vi "Trav_3D_volume.vi"(3 "Simulate/Run":T1, 5 "Traverse line":T2 {"Row Duration (mins)" format="%#.1f"; "Row No" min=0; "Trace Gas Concentration (%)" min=0.0 format="%#.2f"; "Emission Rate (l/min)" format="%#.2f"; "Tunnel Speed" format="%#.2f"; "Start X" format="%#.2f"; "Start Y" format="%#.2f"; "Start Z" format="%#.2f"; "End X" format="%#.2f"; "End Y" format="%#.2f"; "End Z" format="%#.2f"; "Averaging time (min)" min=0.0 format="%#.2f"}) -> (0 "Error Messages":string, 1 "Status":T5, 2 "Traverse line Out":T2 {"Row Duration (mins)" format="%#.1f"; "Row No" min=0; "Trace Gas Concentration (%)" min=0.0 format="%#.2f"; "Emission Rate (l/min)" format="%#.2f"; "Tunnel Speed" format="%#.2f"; "Start X" format="%#.2f"; "Start Y" format="%#.2f"; "Start Z" format="%#.2f"; "End X" format="%#.2f"; "End Y" format="%#.2f"; "End Z" format="%#.2f"; "Averaging time (min)" min=0.0 format="%#.2f"})   [LabVIEW 2011]
uses:
  Gen Trav/Multi_Run_Status.ctl
  Gen Trav/Traverse_cluster.ctl
  Gen Trav/Spacing.ctl
  Controls/Multi_run_mode.ctl
  Controls/User_Specific_mode.ctl
  Controls/Save_Data.ctl
  Controls/Setup.ctl
  ADAM Client/Sub VIs/ADAM Controls/Traverse_Level_State.ctl
  Controls/Overhead.ctl
  Globals/Trav_pos_global.vi
  Globals/Meas_global.vi
panel:
  out "Pause message":string
  in  "Pause":bool
  out "Current position":dbl[](array[numeric]) format="%.2f"
  in  "stop":bool
  in  "Array of Positions":dbl[][](array[numeric]) format="%.2f"
  out "Abcissa copy":string="Y (mm)"
  out "Abcissa":string="Y (mm)"
  in  "Plot 1":i32[](listbox)=[1]
  out "Started Profile at:":string="16/9/98 12:33"
  out "Currently on point":i32=9
  out "U":cluster{dbl[], dbl[]}[](graph)
  out "% u'/U":cluster{dbl[], dbl[]}[](graph)
  # "X           Y            Z"
  # "Start"
  # "End"
  # "X           Y            Z"
  # "Start"
  # "End"
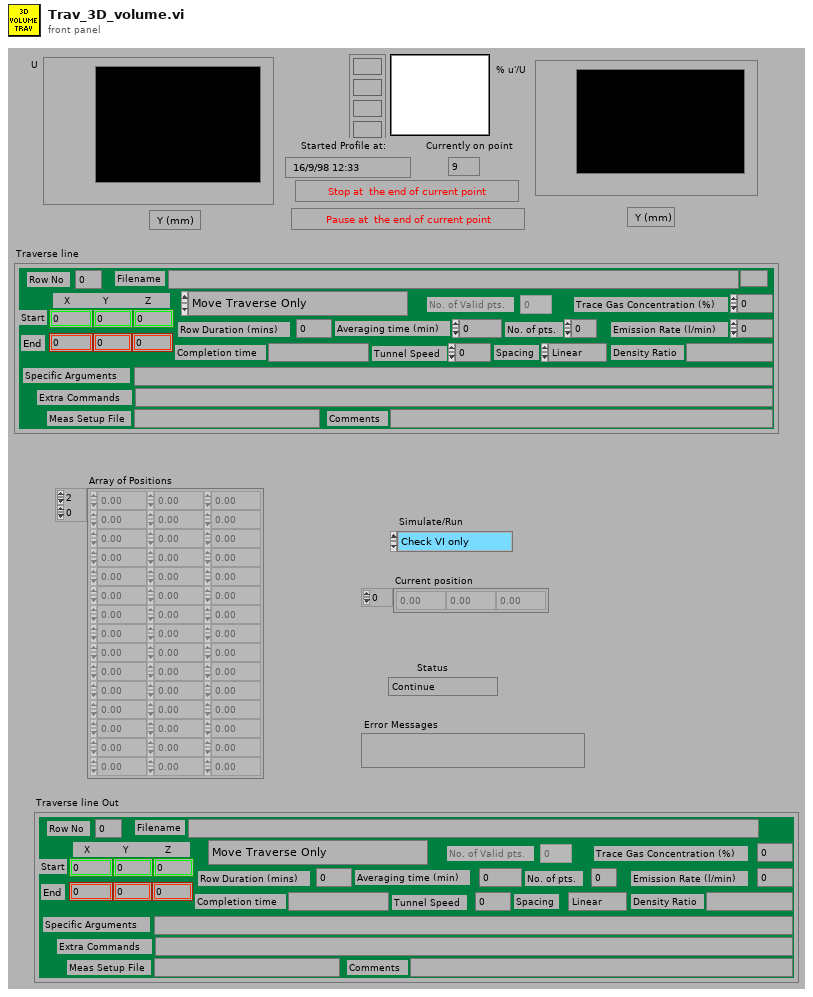
[diagram p1: front panel]
types:
  T1 = typedef "User_Specific_mode.ctl" = enum16{"Check VI only", "Run VI"}
  T2 = typedef "Traverse_cluster.ctl" = cluster{"Start X":dbl, "Start Y":dbl, "Start Z":dbl, "End X":dbl, "End Y":dbl, "End Z":dbl, "No. of pts.":i32, "Spacing":T3, "Filename":path, "Tunnel Speed":dbl, "Averaging time (min)":dbl, "Extra Commands":string, "Specific Arguments":string, "Emission Rate (l/min)":dbl, "Trace Gas Concentration (%)":dbl, "Density Ratio":string, "Comments":string, "Row No":i32, "Row Type Selector":T4, "Completion time":string, "Row Duration (mins)":dbl, "No. of Valid pts.":i32, "Meas Setup File":string}
  T3 = typedef "Spacing.ctl" = enum16{"Linear", "Log", "Gauss", "Specified", "N/A"}
  T4 = typedef "Multi_run_mode.ctl" = enum16{"Move Traverse Only", "Set Tunnel Speed Only", "Set Source Only", "Set Measurement Conditions", "Single Measurement", "Vertical Profile", "Lateral Profile", "Longitudinal Profile", "Explore Volume", "Multi-Axis Profile", "Auto Calibrate", "Meas Fast FID Bkgnd", "Check Beam Power", "Scanning Valve Measurement", "Run VI Named:", "Set ADAM Ch", "Wait (minutes)", "Send Message", "Synchronize With:", "Fall Back to this Row", "Turn Off Row Repeating", "Blank Row", "Traverse 3D Volume"}
  T5 = typedef "Multi_Run_Status.ctl" = enum16{"Continue", "Jump to Next Point", "Jump to Next Row", "Jump To Fall Back", "Terminate Run"}
  T6 = typedef "Save_Data.ctl" = enum16{"Save No Data", "Save Data"}
  T7 = typedef "Setup.ctl" = enum16{"Run Program", "Show Setup", "Save Current Setup", "Setup Front Panel"}
  T8 = typedef "Traverse_Level_State.ctl" = enum16{"Running", "Complete"}
  T9 = typedef "Overhead.ctl" = enum16{"Update total times", "Read Current Overhead", "Re Scale totals to 3 hrs", "Initialise totals to 3hr"}
  T10 = typedef "Status_Cluster.ctl" = cluster{"Status":T5, "Error Type":string, "Error Description":string}
  T11 = typedef "Analysis_info_cluster.ctl" = cluster{"Colour":u32, "Inst type":T12, "Inst name":string, "Symbol":string, "Code name":string, "Extra Info":string, "Inst Array":T13, "Extra Titles":string[], "Extra Values":string[], "Eng Values":dbl[], "Time (ms)":dbl[], "Voltage":dbl[], "U":dbl, "u^2":dbl, "u^3":dbl, "u^4":dbl, "Skew_u":dbl, "Kurt_u":dbl, "Sd Error in Mean":dbl, "% u'/U":dbl, "X":dbl, "Y":dbl, "Z":dbl, "Spectra":T14, "Autocorrelation":T14, "Timescale integral to 25%":dbl, "Sd Error in Variance":dbl, "Calib File":path, "Calib Constants":dbl[], "Histogram":T14, "Output Position":bool, "Full Stats":bool, "Weighting":dbl[], "Av Sampling Rate":dbl, "Av No of Samples":dbl, "Total Meas Time (s)":dbl, "ADAM Ch Name":string}
  T12 = typedef "Inst_type.ctl" = enum16{"Propeller anemometer", "Raw voltage", "Pressure Transducer", "Pitot-static tube", "Preston tube", "Hot wire", "Cross wire 1", "Cross wire 2", "Generic Linear", "Generic Polynomial", "Generic BackPoly", "Fast FID", "Thermocouple", "Cold wire", "Pulsed Wire", "LDA Vel", "LDA Tran time", "LDA Arr time"}
  T13 = typedef "Instrument_Array.ctl" = enum16{"PWA", "LDA", "Analogue"}
  T14 = typedef "XY_Plot_Cluster.ctl" = cluster{"First Name":string, "Second Name":string, "X axis name":string, "Y axis name":string, "X array":dbl[], "Y array":dbl[]}
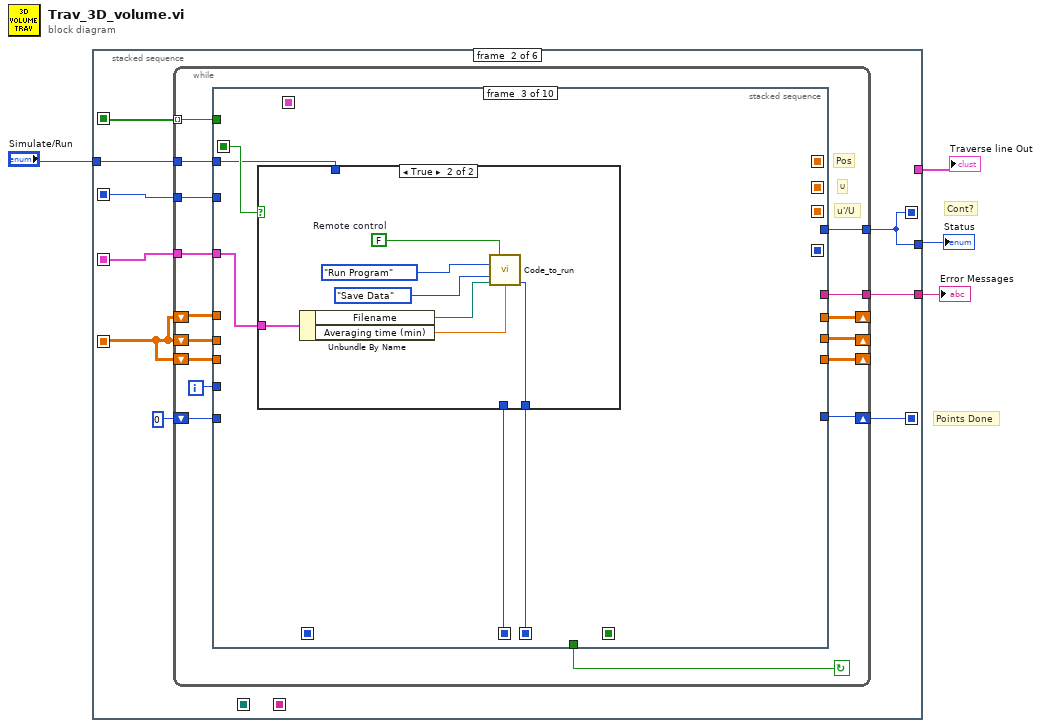
[diagram p0: block diagram]
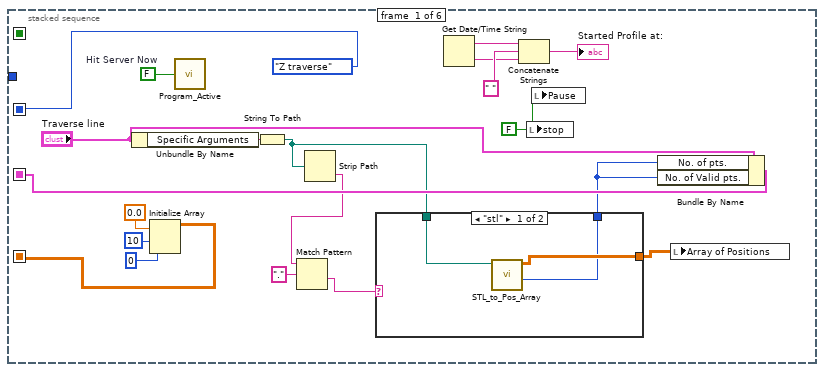
[diagram p2: hidden frame]
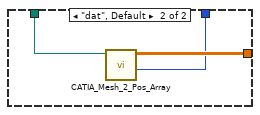
[diagram p3: hidden frame]
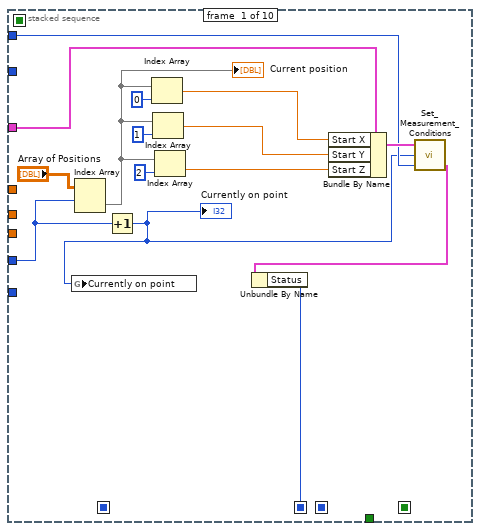
[diagram p4: hidden frame]
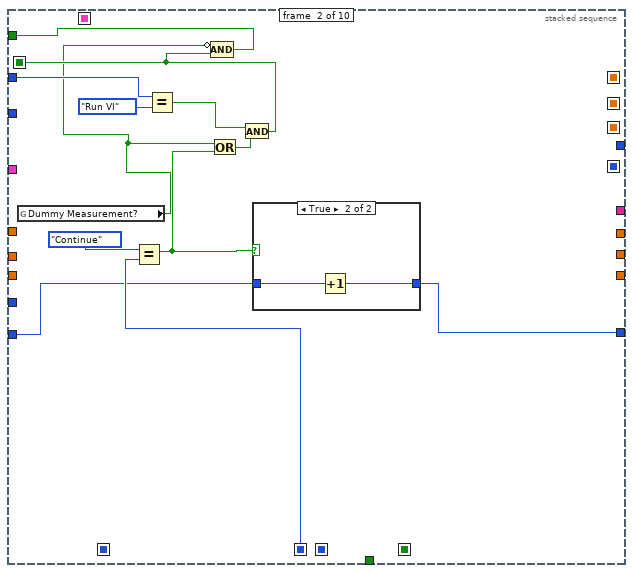
[diagram p5: hidden frame]
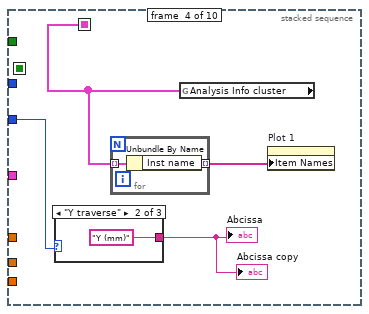
[diagram p8: hidden frame]
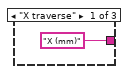
[diagram p9: hidden frame]
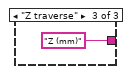
[diagram p10: hidden frame]
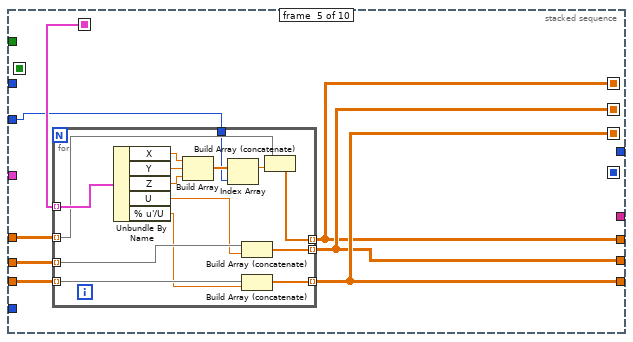
[diagram p11: hidden frame]
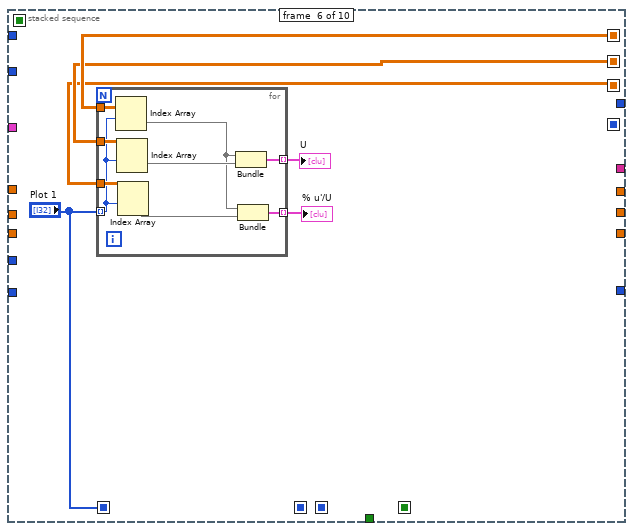
[diagram p12: hidden frame]
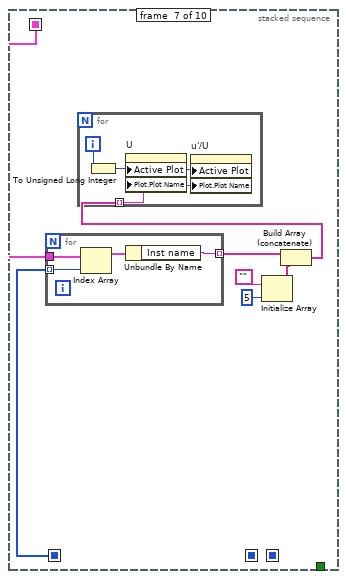
[diagram p13: hidden frame]
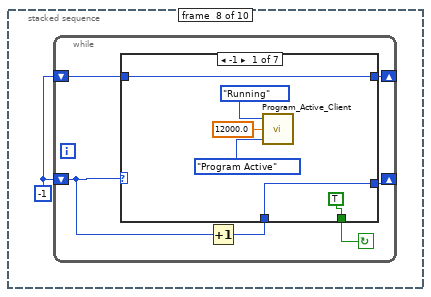
[diagram p14: hidden frame]
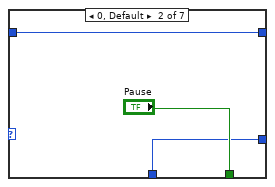
[diagram p15: hidden frame]
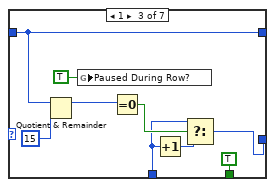
[diagram p16: hidden frame]
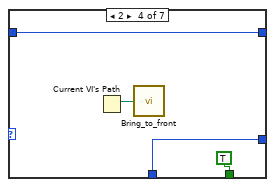
[diagram p17: hidden frame]
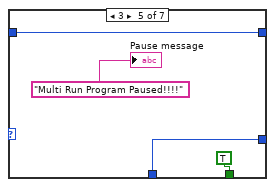
[diagram p18: hidden frame]
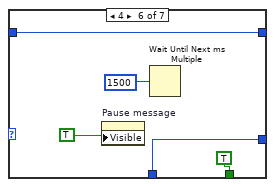
[diagram p19: hidden frame]
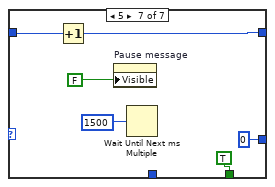
[diagram p20: hidden frame]
diagram:
  # "Points Done"
  # "Cont?"
  n1 = stacked-sequence {
    seq-local: [w17 _ _ _ _ _] -> [_ w38 _ _ _ _]
    seq-local: [enum16{"X traverse", "Y traverse", "Z traverse"}."Z traverse" ("Axis Traversed") _ _ _ _ _] -> [_ w39 _ _ _ _]
    seq-local: [_ _ w264 _ _ _] -> [_ _ _ _ w288 _]
    seq-local: [_ _ _ w271 _ _] -> [_ _ _ _ w287 _]
    seq-local: [_ w37 _ _ _ _] -> [_ _ _ _ _ _]
    seq-local: [_ w35 _ _ _ _] -> [_ _ _ w268 w286 _]
    seq-local: [_ w33 _ _ _ _] -> [_ _ _ _ _ w293]
    seq-local: [w10 _ _ _ _ _] -> [_ w32 _ _ _ w295]
    tunnel: [_ w37 _ _ _ _] -> w2
    tunnel: [_ _ _ _ _ w305] -> w4
    tunnel: "Simulate/Run" -> [_ w36 _ _ _ w304]
    tunnel: [_ w31 _ _ _ _] -> w1
    frame #0 {
      w15 = FALSE ("stop")
      w16 = FALSE  # Hit Server Now
      n2 = Unbundle By Name("Traverse line") -> ("Specific Arguments"=w12:string)
      n3 = Initialize Array(0.0, 10, 0) -> (w17:dbl[][])
      n4 = call "Program_Active.vi"("Hit Server Now"=w16) -> ()
      n5 = String To Path(string=w12) -> (path=w8:path)
      n6 = Strip Path(path=w8) -> (name=w6:string)  [unwired: 1 out]
      n7 = Match Pattern(string=w6, regular expression=".") -> (after substring=w5:string)  [unwired: 1 in, 3 out]
      n8 = case shown="\"stl\"" w5 {
        tunnel: [w26 w30] -> w13
        tunnel: [w25 w29] -> w9
        tunnel: w8 -> [w27 w28]
        frame "stl" {
          n9 = call "STL_to_Pos_Array.vi"("STL file"=w27) -> ("Number of Points"=w25:i32, "Array of Positions"=w26:dbl[][])  [unwired: 9 in]
        }
        frame "dat", Default {
          n10 = call "CATIA_Mesh_2_Pos_Array.vi"("Catia Mesh File"=w28) -> ("Number of Points"=w29:i32, "Array of Positions"=w30:dbl[][])  [unwired: 9 in]
        }
      }
      n11 = Get Date/Time String() -> (date string=w23:string, time string=w22:string)  [unwired: 3 out]
      n12 = Concatenate Strings(w23, " ", w22) -> (→"Started Profile at:":string)
      n13 = local write "stop"(w15) -> ()
      n14 = local write "Pause"(w15) -> ()
      n15 = Bundle By Name(cluster="Traverse line", "No. of pts."=w9, "No. of Valid pts."=w9) -> (w10:T2)
      n16 = local write "Array of Positions"(w13) -> ()
    }
    frame #1 {
      n17 = while {
        shift-left: 0 -> [w42]
        shift-right: [w41] -> w33
        tunnel: [w43] -> w35 mode=indexing
        tunnel: w32 -> [w44]
        tunnel: w36 -> [w45]
        tunnel: [w46] -> w37
        shift-left: w38 -> [w49]
        shift-right: [w48] -> _
        tunnel: w39 -> [w50]
        shift-left: w38 -> [w52]
        shift-right: [w51] -> _
        shift-left: w38 -> [w54]
        shift-right: [w53] -> _
        tunnel: [w40] -> w31
        i -> [w55]
        stop <- w47 continue-if-true
        # "Pos"
        # "U"
        # "u'/U"
        n18 = stacked-sequence {
          seq-local: [_ _ _ w102 _ _ _ _ _ _] -> [_ _ _ _ w113 _ w146 _ _ _]
          seq-local: [_ _ _ _ w109 _ _ _ _ _] -> [_ _ _ _ _ w136 _ _ _ _]
          seq-local: [_ _ _ _ w111 _ _ _ _ _] -> [_ _ _ _ _ w135 _ _ _ _]
          seq-local: [_ _ _ _ w112 _ _ _ _ _] -> [_ _ _ _ _ w134 _ _ _ _]
          seq-local: [_ _ _ _ _ "Plot 1" _ _ _ _] -> [_ _ _ _ _ _ w152 _ _ _]
          seq-local: [_ _ w89 _ _ _ _ _ _ _] -> [_ _ _ _ _ _ _ _ w210 _]
          seq-local: [w60 _ _ _ _ _ _ _ _ _] -> [_ w80 w87 _ _ _ _ _ _ _]
          seq-local: [_ w73 _ _ _ _ _ _ _ _] -> [_ _ w88 _ _ _ _ _ _ _]
          seq-local: [_ _ _ _ _ _ _ _ w205 _] -> [_ _ _ _ _ _ _ _ _ w226]
          seq-local: [_ _ _ _ _ _ _ _ w204 _] -> [_ _ _ _ _ _ _ _ _ w220]
          tunnel: w55 -> [w57 _ _ _ _ _ _ _ w216 w223]
          tunnel: w54 -> [_ _ _ _ w115 _ _ _ _ _]
          tunnel: [_ _ _ _ w111 _ _ _ _ _] -> w53
          tunnel: w52 -> [_ _ _ _ w114 _ _ _ _ _]
          tunnel: [_ _ _ _ w112 _ _ _ _ _] -> w51
          tunnel: w50 -> [_ _ _ w100 w108 _ _ _ _ _]
          tunnel: w49 -> [_ _ _ _ w110 _ _ _ _ _]
          tunnel: [_ _ _ _ w109 _ _ _ _ _] -> w48
          tunnel: [_ _ _ _ _ _ _ _ w205 _] -> w47
          tunnel: w44 -> [w64 _ w90 _ _ _ _ _ _ w224]
          tunnel: [_ _ _ _ _ _ _ _ _ w222] -> w46
          tunnel: w45 -> [w62 w82 w86 _ _ _ _ _ _ w225]
          tunnel: [_ w72 _ _ _ _ _ _ _ _] -> w43
          tunnel: w42 -> [_ w77 _ _ _ _ _ _ _ _]
          tunnel: [_ w76 _ _ _ _ _ _ _ _] -> w41
          tunnel: [_ _ _ _ _ _ _ _ _ w221] -> w40
          frame #0 {
            n19 = Index Array(array="Array of Positions", index (row)=w57) -> (element=w56:dbl[])  [unwired: 1 in]
            "Current position" <- w56
            n20 = Increment(x=w57) -> (x+1=w59:i32)
            "Currently on point" <- w59
            n21 = global write "Trav_pos_global.vi" "Currently on point"(w59) -> ()
            n22 = Index Array(array=w56, index=0 ("Index")) -> (element=w67:dbl)
            n23 = Index Array(array=w56, index=1 ("Index")) -> (element=w66:dbl)
            n24 = Index Array(array=w56, index=2 ("Index")) -> (element=w65:dbl)
            n25 = Bundle By Name(cluster=w64, "Start X"=w67, "Start Y"=w66, "Start Z"=w65) -> (w63:T2)
            n26 = call "Set_Measurement_Conditions.vi"("Simulate/Run"=w62, "Currently on Point"=w59, "Traverse line"=w63) -> ("Status Cluster"=w61:T10)  [unwired: 2 out]
            n27 = Unbundle By Name(w61) -> ("Status"=w60:T5)
          }
          frame #1 {
            n28 = global read "Trav_pos_global.vi" "Dummy Measurement?"() -> (w71:bool)
            n29 = Equal?(x=Multi_Run_Status."Continue" ("Status"), y=w80) -> (x = y?=w75:bool)
            n30 = Equal?(x=w82, y=User_Specific_mode."Run VI" ("Simulate/Run")) -> (x = y?=w78:bool)
            n31 = Or(x=w71, y=w75) -> (x .or. y?=w74:bool)
            n32 = And(x=w78, y=w74) -> (x .and. y?=w73:bool)
            n33 = Compound Arithmetic op=AND(invert w71, w73) -> (w72:bool)
            n34 = case shown="True" w75 {
              tunnel: w77 -> [w83 w85]
              tunnel: [w83 w84] -> w76
              frame False {
              }
              frame True {
                n35 = Increment(x=w85) -> (x+1=w84:i32)
              }
            }
          }
          frame #2 {
            n36 = case shown="True" w88 {
              tunnel: w90 -> [_ w98]
              tunnel: [w91 w97] -> w89
              tunnel: w87 -> [w91 _]
              tunnel: w86 -> [_ _]
              frame False {
              }
              frame True {
                w96 = FALSE  # Remote control
                n37 = Unbundle By Name(w98) -> ("Filename"=w94:path, "Averaging time (min)"=w95:dbl)
                n38 = call "Code_to_run.vi"("setup"=Setup."Run Program", "Remote control"=w96, "File"=Save_Data."Save Data", "Results Filename"=w94, "Averaging time (min)"=w95) -> ("Status"=w97:T5)  [unwired: 6 in, 4 out]
              }
            }
          }
          frame #3 {
            n39 = case shown="\"Y traverse\"" w100 {
              tunnel: ["X (mm)" "Y (mm)" "Z (mm)"] -> w99
              frame "X traverse" {
              }
              frame "Y traverse" {
              }
              frame "Z traverse" {
              }
            }
            "Abcissa" <- w99
            "Abcissa copy" <- w99
            n40 = global read "Meas_global.vi" "Analysis Info cluster"() -> (w102:T11[])
            n41 = for {
              tunnel: w102 -> [w107] mode=indexing
              tunnel: [w106] -> w101 mode=indexing
              n42 = Unbundle By Name(w107) -> ("Inst name"=w106:string)
            }
            n43 = property on="Plot 1" class="LstBox (strict)"("Item Names"=w101) -> ()  [unwired: 2 in, 2 out]
          }
          frame #4 {
            n44 = for {
              tunnel: w115 -> [w130] mode=indexing
              tunnel: [w128] -> w111 mode=indexing
              tunnel: w114 -> [w127] mode=indexing
              tunnel: [w125] -> w112 mode=indexing
              tunnel: w113 -> [w124] mode=indexing
              tunnel: w110 -> [w123] mode=indexing
              tunnel: [w122] -> w109 mode=indexing
              tunnel: w108 -> [w117]
              n45 = Unbundle By Name(w124) -> ("X"=w121:dbl, "Y"=w120:dbl, "Z"=w119:dbl, "U"=w129:dbl, "% u'/U"=w126:dbl)
              n46 = Build Array(w121, w120, w119) -> (w118:dbl[])
              n47 = Index Array(array=w118, index=w117) -> (element=w116:dbl)
              n48 = Build Array (concatenate)(w130, w129) -> (w128:dbl[])
              n49 = Build Array (concatenate)(w127, w126) -> (w125:dbl[])
              n50 = Build Array (concatenate)(w123, w116) -> (w122:dbl[])
            }
          }
          frame #5 {
            n51 = for {
              tunnel: "Plot 1" -> [w137] mode=indexing
              tunnel: w136 -> [w145]
              tunnel: w135 -> [w144]
              tunnel: w134 -> [w143]
              tunnel: [w139] -> w133 mode=indexing
              tunnel: [w138] -> w132 mode=indexing
              n52 = Index Array(array=w145, index (row)=w137) -> (element=w141:dbl[])  [unwired: 1 in]
              n53 = Index Array(array=w144, index (row)=w137) -> (element=w142:dbl[])  [unwired: 1 in]
              n54 = Index Array(array=w143, index (row)=w137) -> (element=w140:dbl[])  [unwired: 1 in]
              n55 = Bundle(w141, w142) -> (w138:cluster{dbl[], dbl[]})  [unwired: 1 out]
              n56 = Bundle(w141, w140) -> (w139:cluster{dbl[], dbl[]})  [unwired: 1 out]
            }
            "U" <- w132
            "% u'/U" <- w133
          }
          frame #6 {
            n57 = for {
              tunnel: w152 -> [w156] mode=indexing
              tunnel: w146 -> [w154]
              tunnel: [w153] -> w149 mode=indexing
              n58 = Index Array(array=w154, index=w156) -> (element=w155:T11)
              n59 = Unbundle By Name(w155) -> ("Inst name"=w153:string)
            }
            n60 = Initialize Array("", 5) -> (w148:string[])
            n61 = Build Array (concatenate)(w149, w148) -> (w147:string[])
            n62 = for {
              tunnel: w147 -> [w157] mode=indexing
              i -> [w159]
              n63 = To Unsigned Long Integer(number=w159) -> (unsigned 32bit integer=w158:u32)
              n64 = property on="U" class="XYGraph (strict)"("Active Plot"=w158, "Plot.Plot Name"=w157) -> ()  [unwired: 2 in, 2 out]
              n65 = property on="u'/U" class="XYGraph (strict)"("Active Plot"=w158, "Plot.Plot Name"=w157) -> ()  [unwired: 2 in, 2 out]
            }
          }
          frame #7 {
            w160 = -1
            n66 = while {
              shift-left: w160 -> [w161]
              shift-right: [w162] -> _
              shift-left: w160 -> [w165]
              shift-right: [w166] -> _
              stop <- w163 continue-if-true
              n67 = Increment(x=w165) -> (x+1=w164:i32)
              n68 = case shown="-1" w165 {
                tunnel: [w171 w174 w178 w188 w191 w195 0] -> w166
                tunnel: w164 -> [w171 w174 w180 w188 w191 w195 _]
                tunnel: [TRUE ("Pause") "Pause" TRUE ("Pause") TRUE ("Pause") TRUE ("Pause") TRUE ("Pause") TRUE ("Pause")] -> w163
                tunnel: [w170 w173 w176 w185 w189 w193 w198] -> w162
                tunnel: w161 -> [w170 w173 w176 w185 w189 w193 w199]
                frame -1 {
                  n69 = call "Program_Active_Client.vi"("Mode"=enum16{"Program Active", "Traverse Level State"}."Program Active", "Time till next contact (Sec)"=12000.0, "Traverse level State"=Traverse_Level_State."Running") -> ()  [unwired: 3 out]
                }
                frame 0, Default {
                }
                frame 1 {
                  n70 = Quotient & Remainder(x=w176, y=15) -> (x-y*floor(x/y)=w182:i32)  [unwired: 1 out]
                  n71 = global write "Trav_pos_global.vi" "Paused During Row?"(TRUE ("Paused During Row?")) -> ()
                  n72 = Equal To 0?(x=w182) -> (x = 0?=w181:bool)
                  n73 = Increment(x=w180) -> (x+1=w179:i32)
                  n74 = Select(t=w180, s=w181, f=w179) -> (s? t:f=w178:i32)
                }
                frame 2 {
                  n75 = Current VI's Path() -> (path=w186:path)
                  n76 = call "Bring_to_front.vi"("path"=w186) -> ()
                }
                frame 3 {
                  "Pause message" <- "Multi Run Program Paused!!!!" ("Pause message")
                }
                frame 4 {
                  n77 = property on="Pause message" class="Str"("Visible"=TRUE) -> ()  [unwired: 2 in, 2 out]
                  n78 = Wait Until Next ms Multiple(millisecond multiple=u32 1500) -> ()  [unwired: 1 out]
                }
                frame 5 {
                  n79 = Increment(x=w199) -> (x+1=w198:i32)
                  n80 = property on="Pause message" class="Str"("Visible"=FALSE) -> ()  [unwired: 2 in, 2 out]
                  n81 = Wait Until Next ms Multiple(millisecond multiple=u32 1500) -> ()  [unwired: 1 out]
                }
              }
            }
          }
          frame #8 {
            n82 = Increment(x=w216) -> (x+1=w215:i32)
            n83 = local read "Array of Positions"() -> (w206:dbl[][])
            n84 = case shown="\"Jump to Next Point\"" w210 {
              tunnel: [TRUE TRUE FALSE] -> w213
              frame "Continue" {
              }
              frame "Jump to Next Point" {
              }
              frame "Jump to Next Row", Default {
              }
            }
            n85 = Array Size(array=w206) -> (size(s)=w209:i32[])
            n86 = Index Array(array=w209, index=0 ("Index")) -> (element=w207:i32)
            n87 = Less?(x=w215, y=w207) -> (x < y?=w214:bool)
            n88 = Compound Arithmetic op=AND(w213, invert "stop", w214) -> (w205:bool)
            n89 = Select(t=Multi_Run_Status."Terminate Run" ("Status"), s="stop", f=w210) -> (s? t:f=w204:T5)
          }
          frame #9 {
            n90 = case shown="True" w226 {
              tunnel: w225 -> [_ w235]
              tunnel: w224 -> [_ w234]
              tunnel: w223 -> [_ w233]
              tunnel: [w228 w230] -> w222
              tunnel: ["" w229] -> w221
              tunnel: w220 -> [w228 _]
              frame False {
              }
              frame True {
                n91 = case shown="\"Check VI only\"" w235 {
                  tunnel: w234 -> [w251 _]
                  tunnel: w233 -> [w246 _]
                  tunnel: [w236 timestamp(0 s since 1904-01-01)] -> w232
                  frame "Check VI only" {
                    n92 = Increment(x=w246) -> (x+1=w244:i32)
                    n93 = Unbundle By Name(w251) -> ("Averaging time (min)"=w248:dbl)
                    n94 = global read "Trav_pos_global.vi" "Simulation Time"() -> (w238:timestamp)
                    n95 = To Double Precision Float(number=w238) -> (double precision float=w239:dbl)
                    n96 = Multiply(x=60.0, y=w248) -> (x*y=w247:dbl)
                    n97 = Add(x=w247, y=10.0 ("Scalable Time (Sec)")) -> (x+y=w245:dbl)
                    n98 = Multiply(x=w245, y=w244) -> (x*y=w242:dbl)
                    n99 = call "Overhead_Factor.vi"("Mode"=Overhead."Read Current Overhead") -> ("Current Overhead Factor"=w243:dbl)  [unwired: 3 in]
                    n100 = Multiply(x=w243, y=w242) -> (x*y=w240:dbl)
                    n101 = Add(x=w239, y=w240) -> (x+y=w237:dbl)
                    n102 = To Time Stamp(1:w237) -> (0:w236:timestamp)
                  }
                  frame "Run VI" {
                  }
                }
                n103 = call "Run_FFID_Bkgnd.vi"("Simulated Time"=w232, "Run Now?"=FALSE, "Simulate/Run"=w235) -> ("Error Messages"=w229:string, "Status"=w230:T5)  [unwired: 1 out]
              }
            }
          }
        }
      }
    }
    frame #2 {
      n104 = global read "Meas_global.vi" "Start Time of experiment"() -> (w254:dbl)
      n105 = global read "Meas_global.vi" "Raw data file"() -> (w266:path)
      n106 = Strip Path(path=w266) -> (stripped path=w265:path)  [unwired: 1 out]
      n107 = call "Sec_to_date_filename.vi"("seconds"=w254) -> ("Day"=w256:string, "Time"=w257:string)  [unwired: 2 out]
      n108 = Format Into String(format string="Cmd_%s_%s.xls", w256, w257) -> (resulting string=w259:string)  [unwired: 2 in, 1 out]
      n109 = call "Fast_string_Replace.vi"("Replace match with:"="-", "Input String"=w259, "regular expression"=":") -> ("Output String"=w262:string)  [unwired: 2 out]
      n110 = call "Fast_string_Replace.vi"("Replace match with:"="", "Input String"=w262, "regular expression"=" ") -> ("Output String"=w253:string)  [unwired: 2 out]
      n111 = Build Path(base path=w265, name or relative path=w253) -> (appended path=w264:path)
    }
    frame #3 {
      w277 = "\t"
      n112 = local read "Array of Positions"() -> (w270:dbl[][])
      n113 = Number To Fractional String(number=w270, precision (6)=i16 2) -> (F-format string=w269:string[][])  [unwired: 2 out]
      n114 = for {
        tunnel: w269 -> [w282] mode=indexing
        tunnel: w268 -> [w281] mode=indexing
        tunnel: [w279] -> w267 mode=indexing
        n115 = case shown="False" w281 {
          tunnel: ["Unobtainable Position" ""] -> w280
          frame False {
          }
          frame True {
          }
        }
        n116 = Build Array (concatenate)(w282, w280) -> (w279:string[])
      }
      n117 = Concatenate Strings("X", w277, "Y", w277, "Z") -> (w272:string)
      n118 = call "2D_array_to_string.vi"("2D data array"=w267, "Column titles  (separated by tabs)"=w272, "Array title"="Requested positions") -> ("Output string"=w271:string)
    }
    frame #4 {
      n119 = Or Array Elements(Boolean array=w286) -> (logical OR=w285:bool)
      n120 = case shown="True" w285 {
        tunnel: w288 -> [_ w291]
        tunnel: w287 -> [_ w289]
        frame False {
        }
        frame True {
          w290 = FALSE  # Lock File
          w292 = TRUE  # append to file? (new file:F)
          n121 = call "Write_Characters_To_File.vi"("file path (dialog if empty)"=w291, "character string"=w289, "append to file? (new file:F)"=w292, "Lock File"=w290) -> ()  [unwired: 1 in, 4 out]
        }
      }
    }
    frame #5 {
      n122 = local read "Array of Positions"() -> (w297:dbl[][])
      n123 = Array Size(array=w297) -> (size(s)=w299:i32[])
      n124 = Index Array(array=w299, index=0 ("Index")) -> (element=w296:i32)
      n125 = Bundle By Name(cluster=w295, "No. of Valid pts."=w293) -> (w294:T2)
      n126 = Not Equal?(x=w296, y=w293) -> (x != y?=w302:bool)
      n127 = Equal?(x=User_Specific_mode."Run VI" ("Simulate/Run"), y=w304) -> (x = y?=w301:bool)
      n128 = And(x=w301, y=w302) -> (x .and. y?=w300:bool)
      n129 = case shown="False" w300 {
        tunnel: w294 -> [w306 w318]
        tunnel: [w306 w317] -> w305
        tunnel: w293 -> [_ w316]
        frame False {
        }
        frame True {
          w307 = " !!Program added comments"
          n130 = Unbundle By Name(w318) -> ("Comments"=w308:string)
          n131 = Equal To 0?(x=w316) -> (x = 0?=w315:bool)
          n132 = Match Pattern(string=w308, regular expression=w307) -> (match substring=w310:string)  [unwired: 4 out]
          n133 = Select(t=" !!(Row Skipped)", s=w315, f=" !!(Row Partially Skipped)") -> (s? t:f=w311:string)
          n134 = Empty String/Path?(string/path=w310) -> (empty?=w309:bool)
          n135 = case shown="True" w309 {
            tunnel: [w321 w325] -> w312
            tunnel: w311 -> [w320 w324]
            tunnel: w307 -> [_ w323]
            tunnel: w308 -> [w319 w322]
            frame False {
              n136 = Concatenate Strings(w319, w320) -> (w321:string)
            }
            frame True {
              n137 = Concatenate Strings(w322, w323, w324) -> (w325:string)
            }
          }
          n138 = Bundle By Name(cluster=w318, "Comments"=w312) -> (w317:T2)
        }
      }
    }
  }
  "Status" <- w2
  "Traverse line Out" <- w4
  "Error Messages" <- w1
